vi "Get Active Program.vi"(5 "Preview Height (Source)":i32, 6 "Get Preview Image? (F)":bool, 7 "Preview Width (Source)":i32, 8 "error in (no error)":errorcluster, 11 "OBS in":refnum<class "OBS.lvclass">) -> (0 "error out":errorcluster, 1 "Preview Image":picture, 2 "Program Scene":string, 3 "OBS out":refnum<class "OBS.lvclass">)   [LabVIEW 2022 SP3, in "obs-websocket-lv.lvlib" / "OBS.lvclass"]
uses:
  OBS.lvclass
  GetCurrentProgramScene/GetCurrentProgramScene.lvclass
  C:/dev/illuminatedg/obs-websocket-lv/obs-websocket-lv/Client Message/Client Message.lvclass
  RGetCurrentProgramScene/RGetCurrentProgramScene.lvclass
  C:/dev/illuminatedg/obs-websocket-lv/obs-websocket-lv/Response/Response.lvclass
  RGetSourceScreenshot/RGetSourceScreenshot.lvclass
  GetSourceScreenshot/GetSourceScreenshot.lvclass
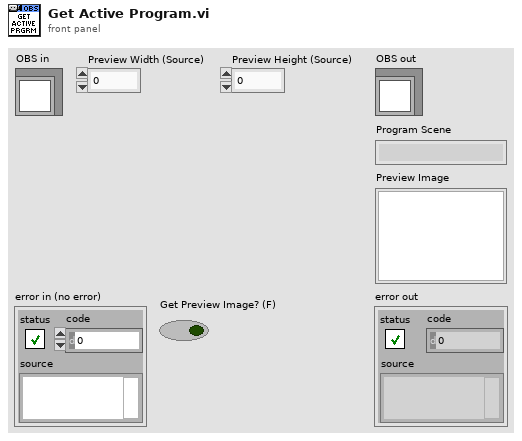
[diagram p1: front panel]
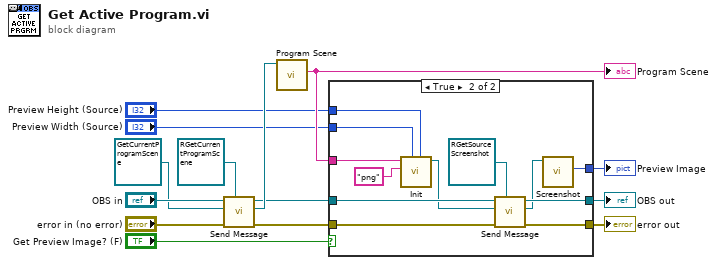
[diagram p0: block diagram]
diagram:
  n1 = call "Send Message.vi"("Response Type (None)"=refnum<class "RGetCurrentProgramScene.lvclass"> refnum ("obs-websocket-lv.lvlib:RGetCurrentProgramScene.lvclass"), "error in (no error)"="error in (no error)", "Client Message"=refnum<class "GetCurrentProgramScene.lvclass"> refnum ("obs-websocket-lv.lvlib:GetCurrentProgramScene.lvclass"), "OBS in"="OBS in") -> ("error out"=w7:errorcluster, "Response"=w10:refnum<class "RGetCurrentProgramScene.lvclass">, "OBS out"=w9:refnum<class "OBS.lvclass">)  [unwired: 4 in, 1 out]
  n2 = call "Program Scene.vi"("RGetCurrentProgramScene in"=w10) -> ("Program Scene"=w6:string)  [unwired: 8 in, 2 out]
  "Program Scene" <- w6
  n3 = case shown="True" "Get Preview Image? (F)" {
    tunnel: w9 -> [w16 w26]
    tunnel: w7 -> [w15 w25]
    tunnel: w6 -> [_ w28]
    tunnel: "Preview Width (Source)" -> [_ w23]
    tunnel: "Preview Height (Source)" -> [_ w22]
    tunnel: [w16 w21] -> w3
    tunnel: [w15 w20] -> w2
    tunnel: [_ w17] -> w1
    frame False {
    }
    frame True {
      n4 = call "Init.vi"("Height (Source)"=w22, "Width (Source)"=w23, "Image Format"="png", "Source Name"=w28) -> ("GetSourceScreenshot out"=w24:refnum<class "GetSourceScreenshot.lvclass">)  [unwired: 6 in, 1 out]
      n5 = call "Send Message.vi"("Response Type (None)"=refnum<class "RGetSourceScreenshot.lvclass"> refnum ("obs-websocket-lv.lvlib:RGetSourceScreenshot.lvclass"), "error in (no error)"=w25, "Client Message"=w24, "OBS in"=w26) -> ("error out"=w20:errorcluster, "Response"=w18:refnum<class "RGetSourceScreenshot.lvclass">, "OBS out"=w21:refnum<class "OBS.lvclass">)  [unwired: 4 in, 1 out]
      n6 = call "Screenshot.vi"("RGetSourceScreenshot in"=w18) -> ("Screenshot"=w17:picture)  [unwired: 8 in, 2 out]
    }
  }
  "error out" <- w2
  "OBS out" <- w3
  "Preview Image" <- w1
